vi "delete_point.vi"(8 "error in (no error)":errorcluster, 10 "point ID":dbl, 11 "PointCollection in":refnum<class "PointCollection.lvclass">) -> (0 "error out":errorcluster, 3 "PointCollection out":refnum<class "PointCollection.lvclass">)   [LabVIEW 2010, in "PointCollection.lvclass"]
uses:
  PointCollection.lvclass
  PointCollection.lvclass/PointCollection.ctl
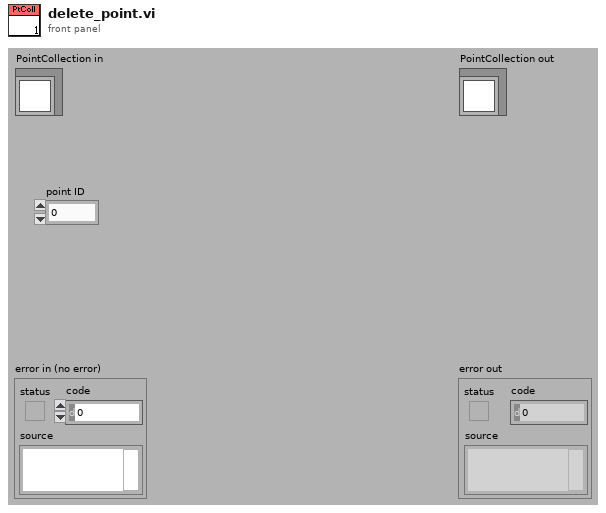
[diagram p1: front panel]
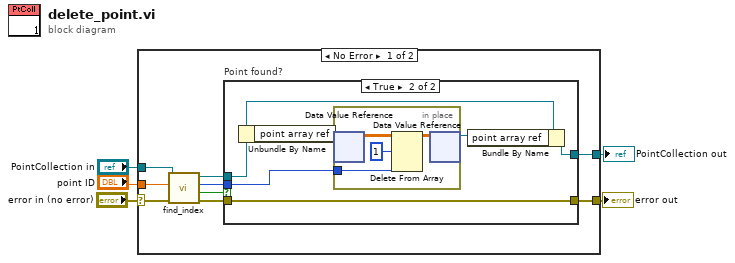
[diagram p0: block diagram]
diagram:
  n1 = case shown="No Error" "error in (no error)" {
    selector: "error in (no error)" -> [w14 w28]
    tunnel: [w6 w28] -> w4
    tunnel: [w10 w27] -> w2
    tunnel: "PointCollection in" -> [w12 w27]
    tunnel: "point ID" -> [w13 _]
    frame No Error {
      n2 = call "find_index.vi"("error in (no error)"=w14, "ID"=w13, "PointCollection in"=w12) -> ("error out"=w7:errorcluster, "found?"=w8:bool, "index"=w11:i32, "PointCollection out"=w9:refnum<class "PointCollection.lvclass">)  [unwired: 5 in]
      n3 = case "Point found?" shown="True" w8 {
        tunnel: w11 -> [_ w21]
        tunnel: [w16 w19] -> w10
        tunnel: w9 -> [w16 w18]
        tunnel: w7 -> [w15 w17]
        tunnel: [w15 w17] -> w6
        frame False {
        }
        frame True {
          n4 = Unbundle By Name(w18) -> ("point array ref"=w22:refnum<data-value>)
          n5 = in-place {
            in-place-border: w21 -> [w23]
            n6 = in-place-dvr #1(w22) -> (w25:dbl[][])  [unwired: 1 out]
            n7 = Delete From Array(array=w25, length=1, index (col)=w23) -> (array with subset deleted=w24:dbl[][])  [unwired: 1 in, 1 out]
            n8 = in-place-dvr #1(w24) -> (w20:refnum<data-value>)  [unwired: 1 out]
          }
          n9 = Bundle By Name(cluster=w18, "point array ref"=w20) -> (w19:refnum<class "PointCollection.lvclass">)
        }
      }
    }
    frame Error {
    }
  }
  "error out" <- w4
  "PointCollection out" <- w2
